vi "Value Multiple Boolean Controls.vi"(8 "error in (no error)":errorcluster, 10 "Enabled":bool, 11 "References":refnum<vi>[](array[refnum])) -> (0 "error out":errorcluster)   [LabVIEW 2015]
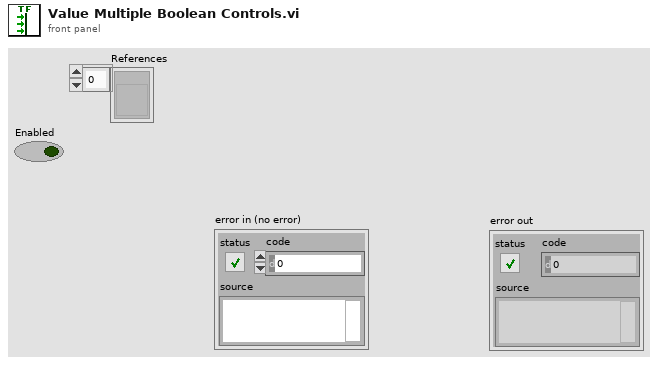
[diagram p1: front panel]
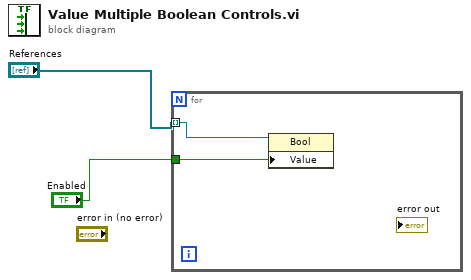
[diagram p0: block diagram]
diagram:
  n1 = for {
    tunnel: "References" -> [w4] mode=indexing
    tunnel: "Enabled" -> [w3]
    n2 = property class="Bool"(reference=w4, "Value"=w3) -> ()  [unwired: 1 in, 2 out]
  }
